vi "DDVL Move Unsed Clusters and Sub Panels.vi"(0 "Cluster Refs":refnum<vi>[](array[refnum]), 11 "Subpanel Refs":refnum<vi>[](array[refnum]), 13 "VI Path/Ref":T1(array[cluster])) -> (4 "Cluster Refs Dup":refnum<vi>[](array[refnum]), 15 "Subpanel Refs Dup":refnum<vi>[](array[refnum]))   [LabVIEW 2016]
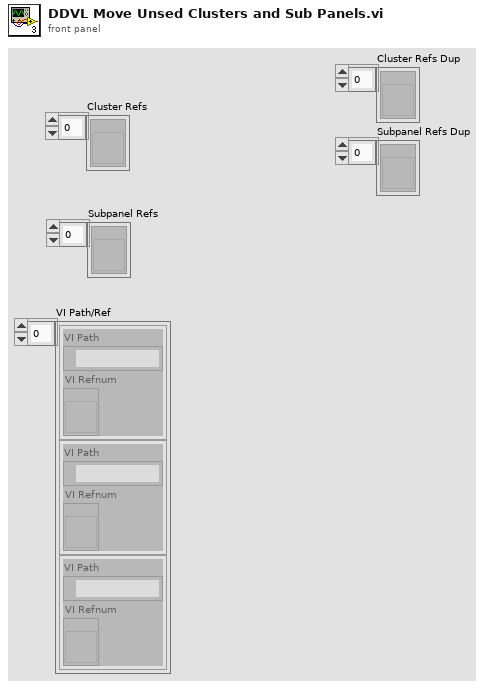
[diagram p1: front panel]
types:
  T1 = cluster{"VI Path":path, "VI Refnum":refnum<vi>}[]
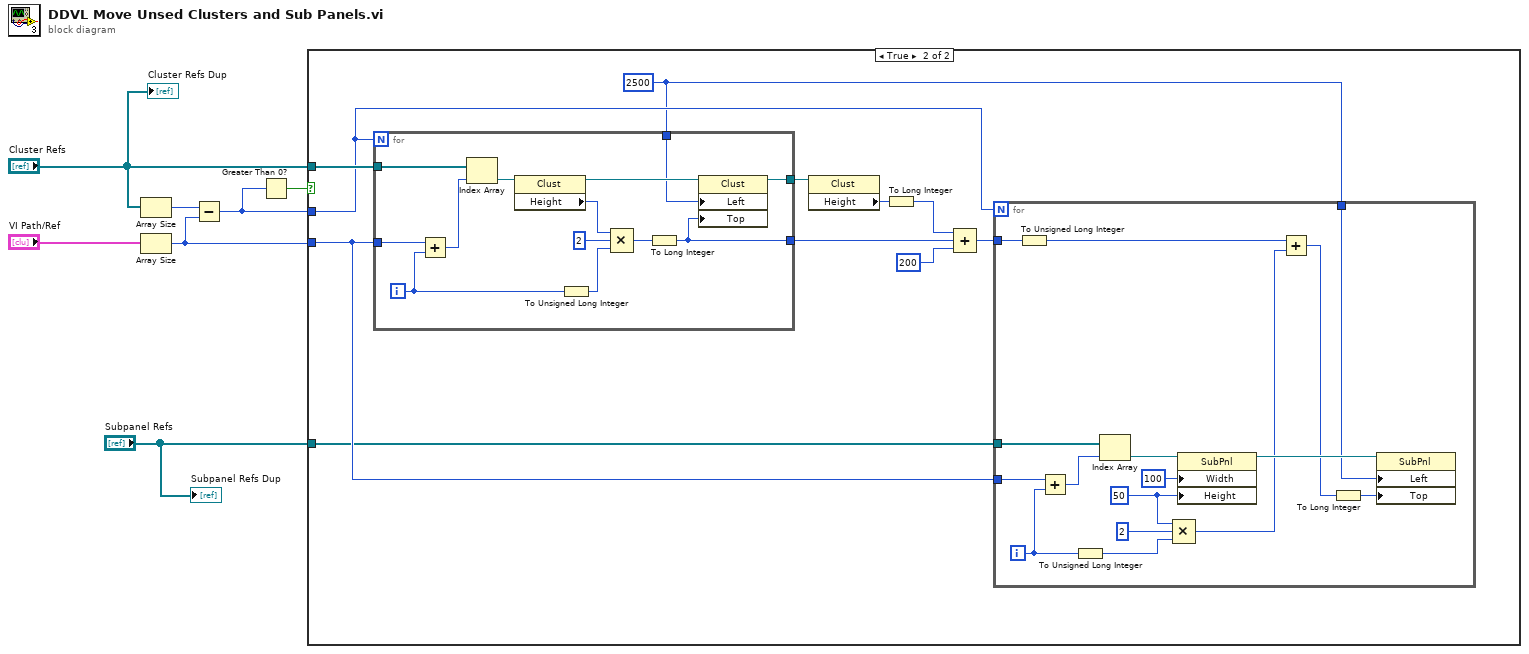
[diagram p0: block diagram]
diagram:
  n1 = Array Size(array="Cluster Refs") -> (size(s)=w6:i32)
  n2 = Array Size(array="VI Path/Ref") -> (size(s)=w4:i32)
  n3 = Subtract(x=w6, y=w4) -> (x-y=w3:i32)
  n4 = Greater Than 0?(x=w3) -> (x > 0?=w2:bool)
  n5 = case shown="True" w2 {
    tunnel: "Cluster Refs" -> [_ w18]
    tunnel: w4 -> [_ w12]
    tunnel: w3 -> [_ w11]
    tunnel: "Subpanel Refs" -> [_ w8]
    frame False {
    }
    frame True {
      w9 = 2500 ("Position:Left")
      n6 = for {
        N: w11 -> [_]
        tunnel: w18 -> [w47]
        tunnel: w12 -> [w46]
        tunnel: [w37] -> w14
        tunnel: [w36] -> w17
        tunnel: w9 -> [w35]
        i -> [w39]
        n7 = Add(x=w46, y=w39) -> (x+y=w38:i32)
        n8 = Index Array(array=w47, index=w38) -> (element=w45:refnum<vi>)
        n9 = property class="Clust"(reference=w45) -> (reference out=w44:refnum<vi>, "Height"=w42:u32)  [unwired: 1 in, 1 out]
        n10 = To Unsigned Long Integer(number=w39) -> (unsigned 32bit integer=w41:u32)
        n11 = Compound Arithmetic op=MULTIPLY(w42, u32 2 ("y"), w41) -> (w40:u32)
        n12 = To Long Integer(number=w40) -> (32bit integer=w37:i32)
        n13 = property class="Clust"(reference=w44, "Left"=w35, "Top"=w37) -> (reference out=w36:refnum<vi>)  [unwired: 1 in, 1 out]
      }
      n14 = property class="Clust"(reference=w17) -> ("Height"=w16:u32)  [unwired: 1 in, 2 out]
      n15 = To Long Integer(number=w16) -> (32bit integer=w15:i32)
      n16 = Compound Arithmetic op=ADD(w15, w14, 200 ("value")) -> (w10:i32)
      n17 = for {
        N: w11 -> [_]
        tunnel: w12 -> [w34]
        tunnel: w8 -> [w33]
        tunnel: w10 -> [w28]
        tunnel: w9 -> [w19]
        i -> [w25]
        w27 = u32 50 ("Container Bounds:Width")
        n18 = To Unsigned Long Integer(number=w28) -> (unsigned 32bit integer=w22:u32)
        n19 = Add(x=w34, y=w25) -> (x+y=w32:i32)
        n20 = To Unsigned Long Integer(number=w25) -> (unsigned 32bit integer=w24:u32)
        n21 = Index Array(array=w33, index=w32) -> (element=w31:refnum<vi>)
        n22 = Compound Arithmetic op=MULTIPLY(w27, u32 2 ("y"), w24) -> (w23:u32)
        n23 = property class="SubPnl"(reference=w31, "Width"=u32 100 ("Container Bounds:Height"), "Height"=w27) -> (reference out=w29:refnum<vi>)  [unwired: 1 in, 1 out]
        n24 = Add(x=w22, y=w23) -> (x+y=w21:u32)
        n25 = To Long Integer(number=w21) -> (32bit integer=w20:i32)
        n26 = property class="SubPnl"(reference=w29, "Left"=w19, "Top"=w20) -> ()  [unwired: 1 in, 2 out]
      }
    }
  }
  "Cluster Refs Dup" <- "Cluster Refs"
  "Subpanel Refs Dup" <- "Subpanel Refs"
